vi "Acquire.vi"(5 "Cluster in":T1={"Queue Array"=[], "Queue Element"={"state"="", "data"=variant}, "System Event"=refnum, "System Event RefNum"=refnum, "Queue List"=[], "LPCA COM"="", "Rotating"=FALSE, "PrecorAI"="", "T_0 Index"=0, "Bar Graph X"=[], "Channels"=[], "Active Indicies"=[], "Active Channels"=[], "Sample Frequency"=0.0, "Ibrake Sweep"=[], "RPM Sweep"=[], "Load Sweep"=[], "Step Height Sweep"=[], "Range Sweep"=[], "A Counter"=0, "B Counter"=0, "C Counter"=0, "#A"=0, "#B"=0, "#C"=0, "Current RPM"=0.0, "Current Ibrake"=0, "Current Range"=0, "Current Step Height"=0, "Load Bank"=enum."OFF", "Cfg Cntrls"=[], "T_Monitor Indices"=[], "Thermal Limit"=0, "Thermal Resume"=0, "Timer Reset"=FALSE, "Stop Time"=0.0, "Autotest"=FALSE, "Pulsed RPM Capture"=FALSE, "Get Sample"=FALSE, "Last State"="", "Reset Timeout"=FALSE, "Ctrl Refs"={"Test Details"=refnum, "Save Config"=refnum, "Load Config"=refnum, "Path"=refnum, "Snapshot"=refnum, "SS#"=refnum, "Ibrake"=refnum, "RPM Target"=refnum, "Spin"=refnum, "Load Bank"=refnum, "Start Test"=refnum, "Pause Test"=refnum, "Load Sweep"=refnum, "RPM Sweep"=refnum, "Ibrake Sweep"=refnum, "Filters"=refnum, "Sample Frequency"=refnum, "Data Setup"=refnum, "Pause"=refnum, "Stop Time"=refnum, "S Period"=refnum, "Range"=refnum, "Step Height"=refnum, "Step Height Sweep"=refnum, "Range Sweep"=refnum, "Available Tests"=refnum, "RPM Graph"=refnum, "RPM Knob"=refnum, "FanMode"=refnum, "Fan Mode LED Array"=refnum, "Thermal Equilibrium"=refnum, "Data Display"=refnum, "LPCA Error"=refnum, "LPCA Ramp"=refnum, "LPCA Range"=refnum, "LPCA Resistance"=refnum, "Analyze Read"=refnum, "Console Select"=refnum, "Sub Panel"=refnum}, "Pulse Waveform"={"t0"=timestamp(0 s since 1904-01-01), "dt"=1.0, "Y"=[]}, "Snapshot"={"Test Details"="test", "Version"="test", "Date"=timestamp(3493915594.3018084 s since 1904-01-01), "Selected Test"="man", "Snapshot Number"=0, "Time"=timestamp(3493915602.7292905 s since 1904-01-01), "Ibrake Setpoint"="1", "RPM Setpoint"="20", "Range Setpoint"="", "Step Height Setpoint"="", "Load Bank Setpoint"="15", "Measurement Headers"="a,b,c,1,2,3", "Measurements"="1,2,3,4,5,6,7,8", "A"=0, "B"=0, "C"=0, "Raw Data"=[], "Available Tests"=enum."Manual", "Ibrake List"="", "RPM List"="", "Load Bank List"="", "Range List"="", "Step Height List"="", "FanMode Setpoint"=enum."Auto"}, "Sample Period"=0.0, "OverTemp"=FALSE, "Available Tests"=enum."Manual", "FanMode"=enum."Auto", "Fan Mode LED Array"=[FALSE, TRUE, FALSE], "Thermal\nEquilibrium "=FALSE, "Equilibrium Stop"=FALSE, "AvgDegChg"=[]} {"Snapshot"."Time" format="%<%H:%M:%S>T"; "Snapshot"."Date" format="%<%m/%d/%Y>T"}, 7 "Filters":T9(ring), 9 "Available Tests":T6, 10 "Active":bool, 11 "error in (no error)":errorcluster, 12 "Snapshot in":bool) -> (1 "output cluster":T1={"Queue Array"=[], "Queue Element"={"state"="", "data"=variant}, "System Event"=refnum, "System Event RefNum"=refnum, "Queue List"=[], "LPCA COM"="", "Rotating"=FALSE, "PrecorAI"="", "T_0 Index"=0, "Bar Graph X"=[], "Channels"=[], "Active Indicies"=[], "Active Channels"=[], "Sample Frequency"=0.0, "Ibrake Sweep"=[], "RPM Sweep"=[], "Load Sweep"=[], "Step Height Sweep"=[], "Range Sweep"=[], "A Counter"=0, "B Counter"=0, "C Counter"=0, "#A"=0, "#B"=0, "#C"=0, "Current RPM"=0.0, "Current Ibrake"=0, "Current Range"=0, "Current Step Height"=0, "Load Bank"=enum."OFF", "Cfg Cntrls"=[], "T_Monitor Indices"=[], "Thermal Limit"=0, "Thermal Resume"=0, "Timer Reset"=FALSE, "Stop Time"=0.0, "Autotest"=FALSE, "Pulsed RPM Capture"=FALSE, "Get Sample"=FALSE, "Last State"="", "Reset Timeout"=FALSE, "Ctrl Refs"={"Test Details"=refnum, "Save Config"=refnum, "Load Config"=refnum, "Path"=refnum, "Snapshot"=refnum, "SS#"=refnum, "Ibrake"=refnum, "RPM Target"=refnum, "Spin"=refnum, "Load Bank"=refnum, "Start Test"=refnum, "Pause Test"=refnum, "Load Sweep"=refnum, "RPM Sweep"=refnum, "Ibrake Sweep"=refnum, "Filters"=refnum, "Sample Frequency"=refnum, "Data Setup"=refnum, "Pause"=refnum, "Stop Time"=refnum, "S Period"=refnum, "Range"=refnum, "Step Height"=refnum, "Step Height Sweep"=refnum, "Range Sweep"=refnum, "Available Tests"=refnum, "RPM Graph"=refnum, "RPM Knob"=refnum, "FanMode"=refnum, "Fan Mode LED Array"=refnum, "Thermal Equilibrium"=refnum, "Data Display"=refnum, "LPCA Error"=refnum, "LPCA Ramp"=refnum, "LPCA Range"=refnum, "LPCA Resistance"=refnum, "Analyze Read"=refnum, "Console Select"=refnum, "Sub Panel"=refnum}, "Pulse Waveform"={"t0"=timestamp(0 s since 1904-01-01), "dt"=1.0, "Y"=[]}, "Snapshot"={"Test Details"="test", "Version"="test", "Date"=timestamp(3493915594.3018084 s since 1904-01-01), "Selected Test"="man", "Snapshot Number"=0, "Time"=timestamp(3493915602.7292905 s since 1904-01-01), "Ibrake Setpoint"="1", "RPM Setpoint"="20", "Range Setpoint"="", "Step Height Setpoint"="", "Load Bank Setpoint"="15", "Measurement Headers"="a,b,c,1,2,3", "Measurements"="1,2,3,4,5,6,7,8", "A"=0, "B"=0, "C"=0, "Raw Data"=[], "Available Tests"=enum."Manual", "Ibrake List"="", "RPM List"="", "Load Bank List"="", "Range List"="", "Step Height List"="", "FanMode Setpoint"=enum."Auto"}, "Sample Period"=0.0, "OverTemp"=FALSE, "Available Tests"=enum."Manual", "FanMode"=enum."Auto", "Fan Mode LED Array"=[FALSE, TRUE, FALSE], "Thermal\nEquilibrium "=FALSE, "Equilibrium Stop"=FALSE, "AvgDegChg"=[]} {"Snapshot"."Time" format="%<%H:%M:%S>T"; "Snapshot"."Date" format="%<%m/%d/%Y>T"}, 3 "Over Temp":bool, 4 "Heartbeat":bool caption="Time has Elapsed", 6 "Parsed Data":T8, 8 "Mean RPM":dbl format="%0.2f", 13 "RPM Wfm":cluster{"X":dbl, "Y":dbl}[](array[cluster]), 14 "Waveform 5 seconds":waveform(dbl)[](array[waveform]), 15 "error out":errorcluster)   [LabVIEW 2017]
uses:
  Controls/Available Tests.ctl
  Controls/Test TypeDef.ctl
  Code Library/Queue References Array.ctl
  Code Library/Queue Element.ctl
  Controls/Load Bank.ctl
  Console Sim/Controls/Console Select.ctl
  Controls/Snapshot Typedef.ctl
  Controls/FanMode.ctl
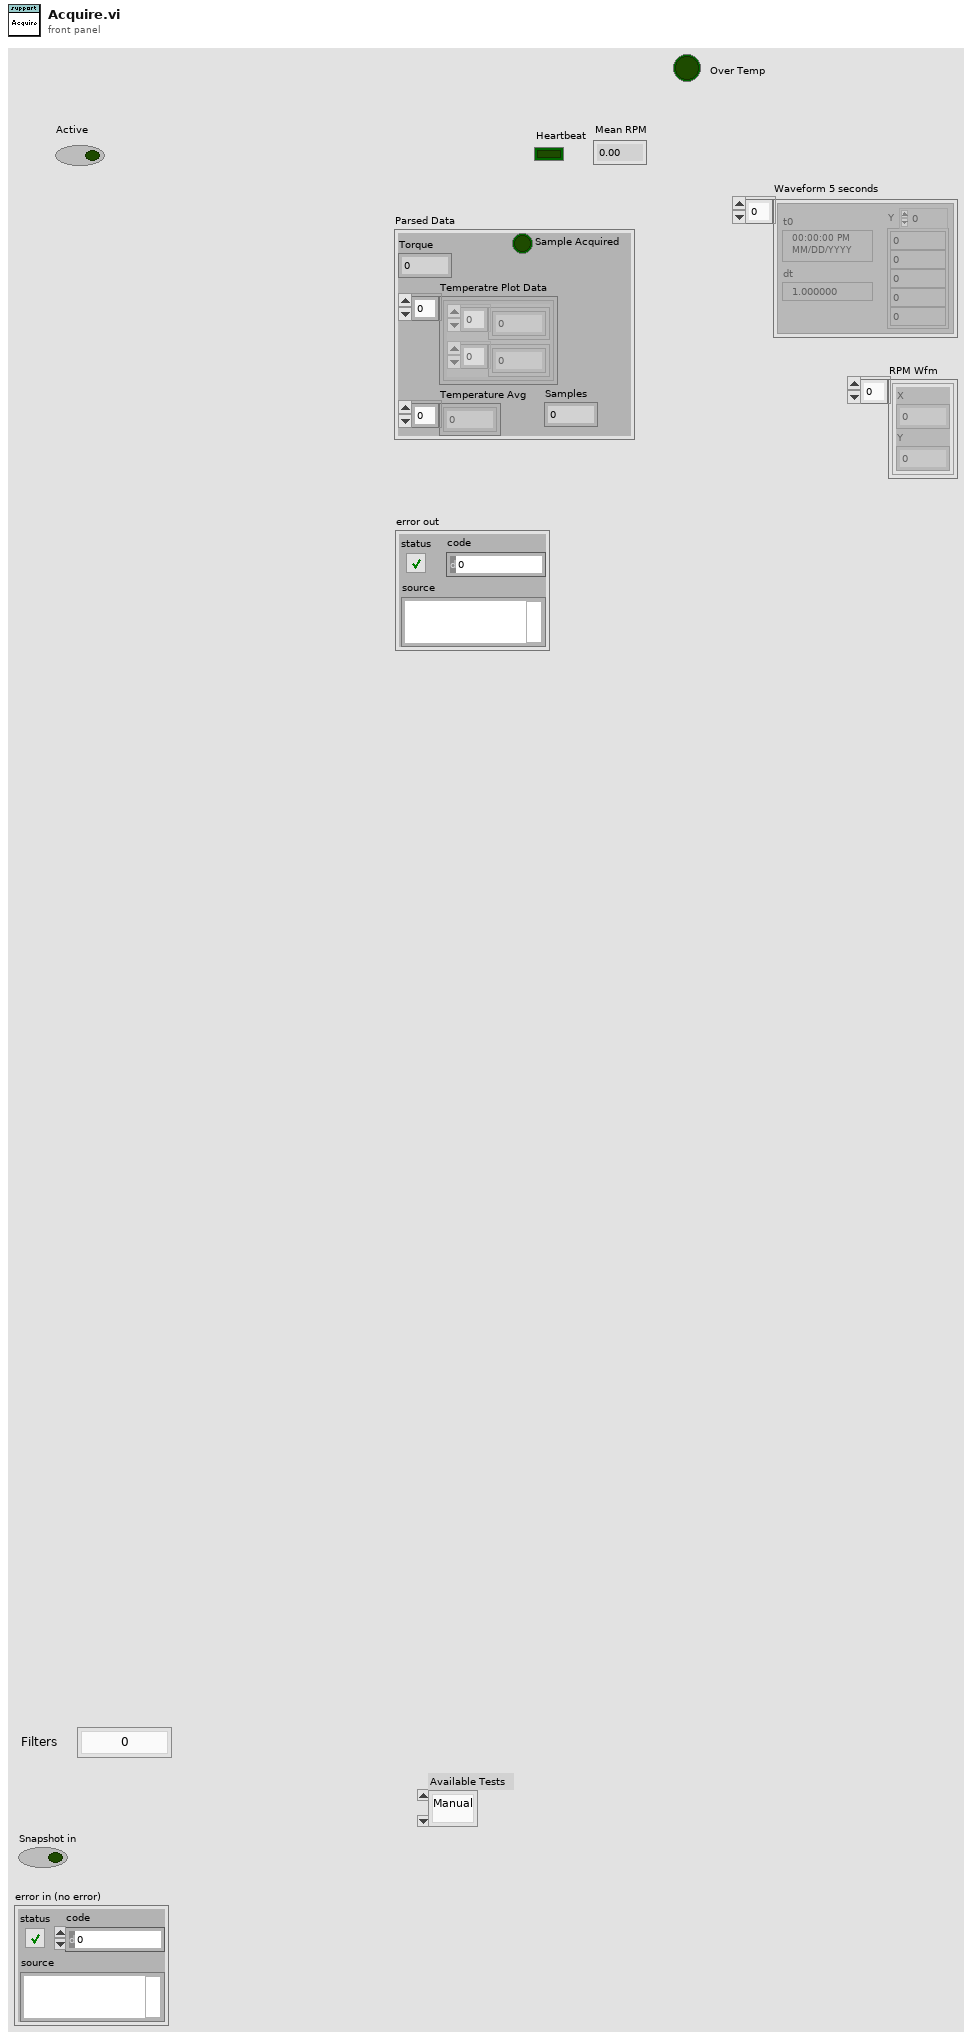
[diagram p1: front panel]
types:
  T1 = typedef "Test TypeDef.ctl" = cluster{"Queue Array":T2, "Queue Element":T3, "System Event":refnum<user-event>, "System Event RefNum":refnum<event-registration>, "Queue List":string[], "LPCA COM":refnum<visa-resource-name>, "Rotating":bool, "PrecorAI":refnum<k21>, "T_0 Index":i32, "Bar Graph X":i32[], "Channels":string[], "Active Indicies":i32[], "Active Channels":string[][], "Sample Frequency":dbl, "Ibrake Sweep":string[], "RPM Sweep":string[], "Load Sweep":string[], "Step Height Sweep":string[], "Range Sweep":string[], "A Counter":i32, "B Counter":i32, "C Counter":i32, "#A":i32, "#B":i32, "#C":i32, "Current RPM":dbl, "Current Ibrake":u32, "Current Range":u32, "Current Step Height":u32, "Load Bank":T4, "Cfg Cntrls":refnum<vi>[], "T_Monitor Indices":i32[], "Thermal Limit":i32, "Thermal Resume":i32, "Timer Reset":bool, "Stop Time":dbl, "Autotest":bool, "Pulsed RPM Capture":bool, "Get Sample":bool, "Last State":string, "Reset Timeout":bool, "Ctrl Refs":cluster{"Test Details":refnum<vi>, "Save Config":refnum<vi>, "Load Config":refnum<vi>, "Path":refnum<vi>, "Snapshot":refnum<vi>, "SS#":refnum<vi>, "Ibrake":refnum<vi>, "RPM Target":refnum<vi>, "Spin":refnum<vi>, "Load Bank":refnum<vi>, "Start Test":refnum<vi>, "Pause Test":refnum<vi>, "Load Sweep":refnum<vi>, "RPM Sweep":refnum<vi>, "Ibrake Sweep":refnum<vi>, "Filters":refnum<vi>, "Sample Frequency":refnum<vi>, "Data Setup":refnum<vi>, "Pause":refnum<vi>, "Stop Time":refnum<vi>, "S Period":refnum<vi>, "Range":refnum<vi>, "Step Height":refnum<vi>, "Step Height Sweep":refnum<vi>, "Range Sweep":refnum<vi>, "Available Tests":refnum<vi>, "RPM Graph":refnum<vi>, "RPM Knob":refnum<vi>, "FanMode":refnum<vi>, "Fan Mode LED Array":refnum<vi>, "Thermal Equilibrium":refnum<vi>, "Data Display":refnum<vi>, "LPCA Error":refnum<vi>, "LPCA Ramp":refnum<vi>, "LPCA Range":refnum<vi>, "LPCA Resistance":refnum<vi>, "Analyze Read":refnum<vi>, "Console Select":refnum<vi>, "Sub Panel":refnum<vi>}, "Pulse Waveform":waveform(dbl), "Snapshot":T5, "Sample Period":dbl, "OverTemp":bool, "Available Tests":T6, "FanMode":T7, "Fan Mode LED Array":bool[], "Thermal\nEquilibrium ":bool, "Equilibrium Stop":bool, "AvgDegChg":dbl[]}
  T2 = typedef "Queue References Array.ctl" = refnum<queue>[]
  T3 = typedef "Queue Element.ctl" = cluster{"state":string, "data":variant}
  T4 = typedef "Load Bank.ctl" = enum16{"OFF", "50", "25", "16.7", "12.5", "10.0", "8.3", "7.1", "6.3", "5.6", "5.0", "4.5", "4.2", "3.8", "3.6", "3.3", "3.1"}
  T5 = typedef "Snapshot Typedef.ctl" = cluster{"Test Details":string, "Version":string, "Date":timestamp, "Selected Test":string, "Snapshot Number":u16, "Time":timestamp, "Ibrake Setpoint":string, "RPM Setpoint":string, "Range Setpoint":string, "Step Height Setpoint":string, "Load Bank Setpoint":string, "Measurement Headers":string, "Measurements":string, "A":i32, "B":i32, "C":i32, "Raw Data":string[][], "Available Tests":T6, "Ibrake List":string, "RPM List":string, "Load Bank List":string, "Range List":string, "Step Height List":string, "FanMode Setpoint":T7}
  T6 = typedef "Available Tests.ctl" = enum16{"Manual", "EFX Brake Torque", "Generator Torque", "EFX Brake Thermal", "Generator Thermal", "Pulsed RPM", "AMT Brake Torque", "Bike Brake Torque", "AMT Brake Thermal", "Bike Brake Thermal"}
  T7 = typedef "FanMode.ctl" = enum16{"On", "Off", "Auto"}
  T8 = cluster{"Sample Acquired":bool, "Torque":dbl, "Temperatre Plot Data":cluster{dbl[], i32[]}[], "Temperature Avg":dbl[], "Samples":i32}
  T9 = enum16{"0", "0.1", "0.2", "0.5", "1", "2", "5", "10", "20", "50", "100", "200", "500", "1000", "2000", "5000", "10000"}
  T10 = cluster{bool, "Torque":dbl, "Temperatre Plot Data":cluster{dbl[], i32[]}[], "Temperature Avg":dbl[], "number of samples per channel":i32}
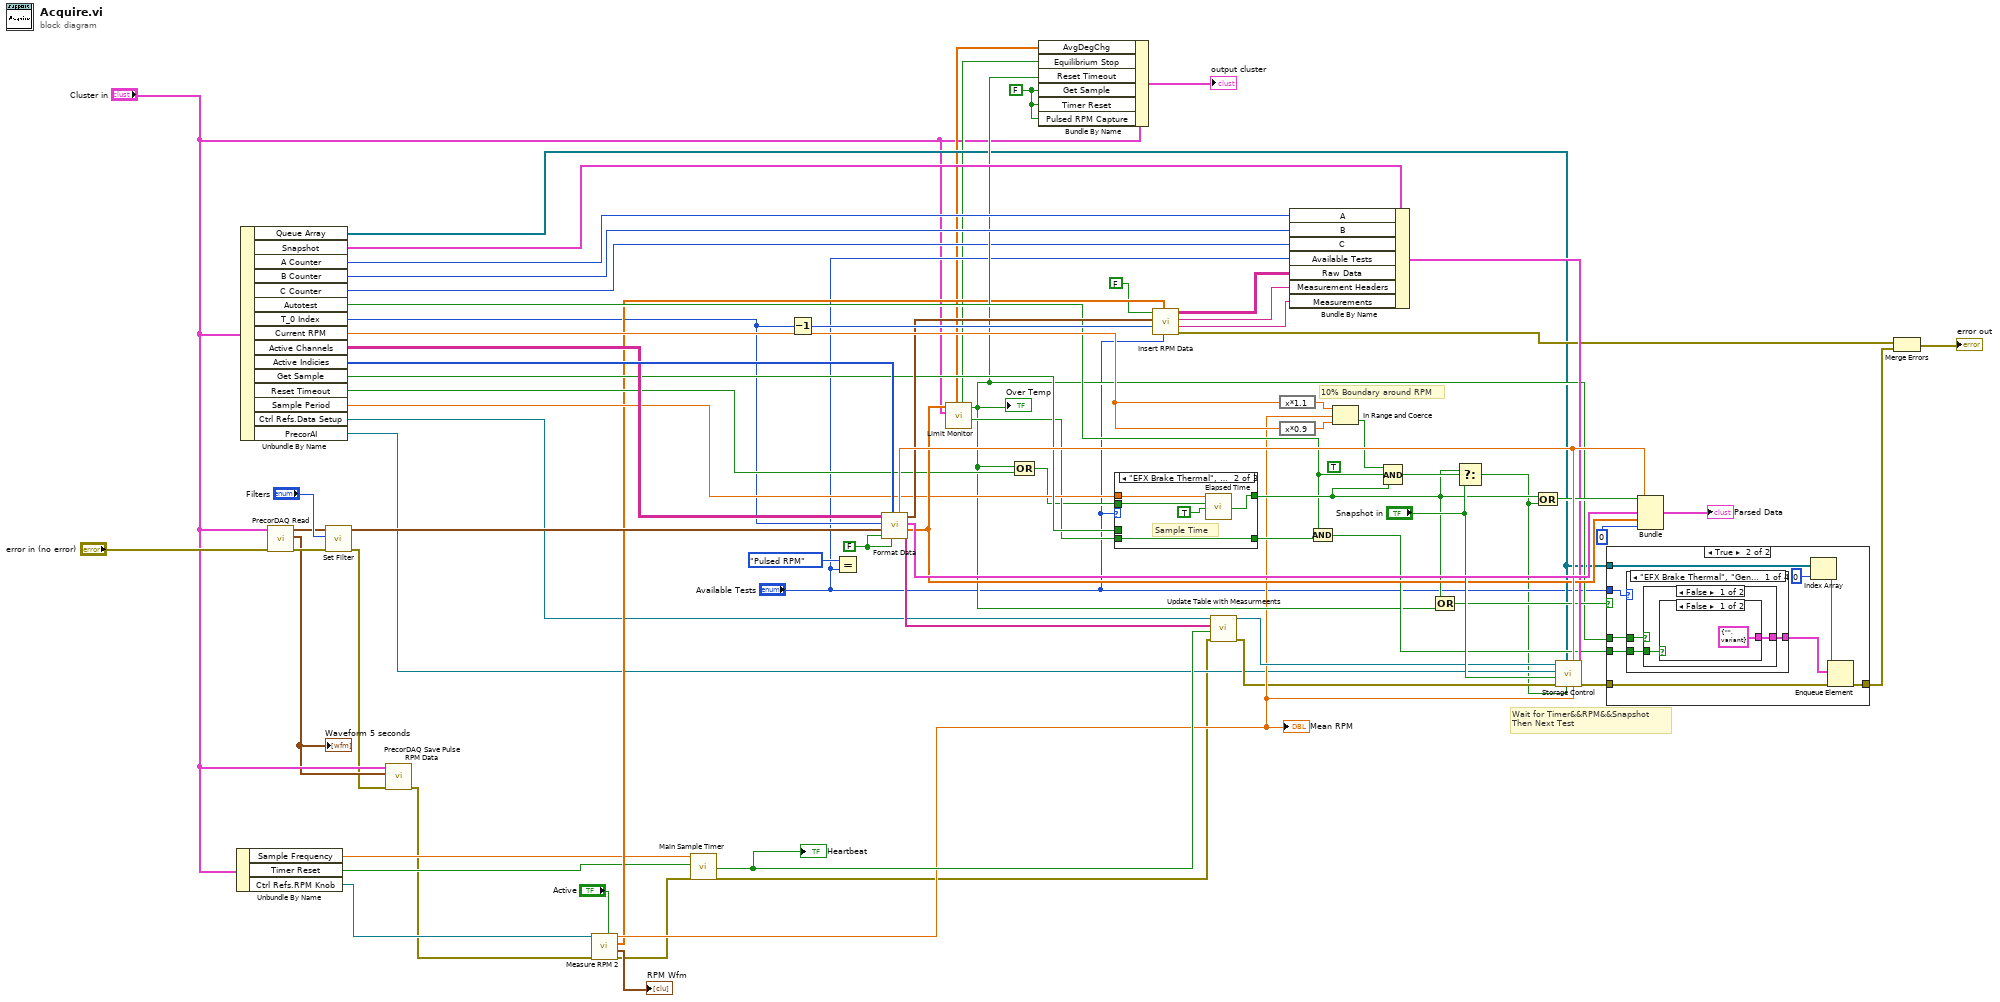
[diagram p0: block diagram]
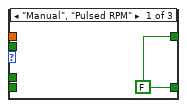
[diagram p2: hidden frame]
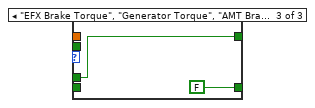
[diagram p3: hidden frame]
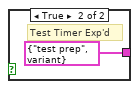
[diagram p5: hidden frame]
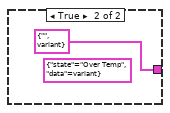
[diagram p6: hidden frame]
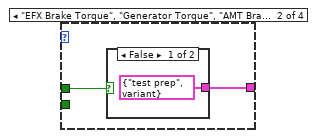
[diagram p7: hidden frame]
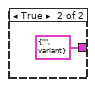
[diagram p8: hidden frame]
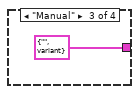
[diagram p9: hidden frame]
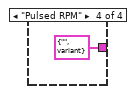
[diagram p10: hidden frame]
diagram:
  (unwired) TRUE ("value")
  w2 = FALSE ("Reset")
  w8 = FALSE
  # "10% Boundary around RPM"
  # "Wait for Timer&&RPM&&Snapshot\nThen Next Test"
  n1 = Unbundle By Name("Cluster in") -> ("Sample Frequency"=w11:dbl, "Timer Reset"=w12:bool, "Ctrl Refs.RPM Knob"=w16:refnum<vi>)
  n2 = Unbundle By Name("Cluster in") -> ("Queue Array"=w25:T2, "Snapshot"=w45:T5, "A Counter"=w56:i32, "B Counter"=w57:i32, "C Counter"=w33:i32, "Autotest"=w37:bool, "T_0 Index"=w22:i32, "Current RPM"=w65:dbl, "Active Channels"=w67:string[][], "Active Indicies"=w71:i32[], "Get Sample"=w50:bool, "Reset Timeout"=w36:bool, "Sample Period"=w43:dbl, "Ctrl Refs.Data Setup"=w28:refnum<vi>, "PrecorAI"=w13:refnum<k21>)
  n3 = call "PrecorDAQ Read.vi"("error in (no error)"="error in (no error)", "Cluster"="Cluster in") -> ("error out"=w15:errorcluster, "Data 5 seconds"=w6:waveform(dbl)[], "Data"=w14:waveform(dbl)[])  [unwired: 7 in]
  "Waveform 5 seconds" <- w6
  n4 = call "Set Filter.vi"("error in (no error)"=w15, "Filters"="Filters", "data"=w14) -> ("error out"=w5:errorcluster, "Array of Waveform"=w54:waveform(dbl)[])  [unwired: 7 in]
  n5 = call "PrecorDAQ Save Pulse RPM Data.vi"("error in (no error)"=w5, "Pulse RPM Data"=w6, "Cluster"="Cluster in") -> ("error out"=w4:errorcluster)  [unwired: 8 in]
  n6 = call "Measure RPM 2.vi"("Active"="Active", "error in"=w4, "Knob in"=w16) -> ("error out"=w10:errorcluster, "RPM Wfm"=→"RPM Wfm":cluster{"X":dbl, "Y":dbl}[], "Raw"=w30:dbl[], "Median RPM"=w31:dbl)  [unwired: 5 in]
  "Mean RPM" <- w31
  n7 = call "Main Sample Timer"("Time Target (s)"=w11, "Reset"=w12, "error in (no error)"=w10) -> ("Time has Elapsed"=w51:bool, "error out"=w9:errorcluster)  [unwired: 9 in, 6 out]
  "Heartbeat" <- w51
  n8 = Decrement(x=w22) -> (x-1=w55:i32)
  n9 = Equal?(x=Available_Tests."Pulsed RPM", y="Available Tests") -> ()  [unwired: 1 out]
  n10 = call "Format Data.vi"("Raw?"=w2, "Inidicies"=w71, "Reset"=w2, "data"=w54, "T_0 Index"=w22, "Active Channels"=w67) -> ("AI Chan Avg."=w68:string[], "Temperature Avg"=w61:dbl[], "Temperatre Plot Data"=w74:cluster{dbl[], i32[]}[], "Data Out"=w53:waveform(dbl)[], "Torque"=w62:dbl)  [unwired: 1 out]
  n11 = call "Limit Monitor.vi"("Cluster"="Cluster in", "Temperature Avg"=w61) -> ("Test Timer"=w41:bool, "Over Temp"=w34:bool, "Equilibrium Stop"=w20:bool, "AvgDegChg"=w19:dbl[])  [unwired: 6 in]
  "Over Temp" <- w34
  n12 = Compound Arithmetic op=OR(w34, w36) -> (w35:bool)
  n13 = Bundle By Name(cluster="Cluster in", "AvgDegChg"=w19, "Equilibrium Stop"=w20, "Reset Timeout"=w34, "Get Sample"=w8, "Timer Reset"=w8, "Pulsed RPM Capture"=w8) -> (→"output cluster":T1)
  n14 = case shown="\"EFX Brake Thermal\", \"Generator Thermal\", \"AMT Brake Thermal\", \"Bike Brake Thermal\"" "Available Tests" {
    tunnel: [w75 w79 w82] -> w42
    tunnel: w50 -> [_ _ w82]
    tunnel: w35 -> [_ w76 _]
    tunnel: w43 -> [_ w78 _]
    tunnel: w41 -> [_ w77 _]
    tunnel: [w75 w77 FALSE ("Test Timer")] -> w39
    frame "Manual", "Pulsed RPM" {
      w75 = FALSE ("Test Timer")
    }
    frame "EFX Brake Thermal", "Generator Thermal", "AMT Brake Thermal", "Bike Brake Thermal" {
      # "Sample Time"
      n15 = call "Elapsed Time"("Time Target (s)"=w78, "Reset"=w76, "Auto Reset"=TRUE) -> ("Time has Elapsed"=w79:bool)  [unwired: 9 in, 7 out]
    }
    frame "EFX Brake Torque", "Generator Torque", "AMT Brake Torque", "Bike Brake Torque" {
    }
  }
  n16 = call "Insert RPM Data.vi"("Available Tests"="Available Tests", "Raw"=w30, "Numeric"=w55, "Data Out in"=w53, "Pulsed RPM Capture"=FALSE) -> ("error out"=w52:errorcluster, "Measurements"=w23:string, "Header"=w26:string, "Data Out out"=w24:string[][])  [unwired: 2 in, 1 out]
  n17 = call "Update Table with Measurmeents.vi"("error in (no error)"=w9, "Sample"=w51, "AI Chan Avg."=w68, "MulticolumnListbox in"=w28) -> ("error out"=w27:errorcluster, "MulticolumnListbox out"=w69:refnum<vi>)  [unwired: 6 in]
  n18 = expression code="x*1.1"(w65) -> (w63:dbl)
  n19 = expression code="x*0.9"(w65) -> (w64:dbl)
  n20 = Bundle By Name(cluster=w45, "A"=w56, "B"=w57, "C"=w33, "Available Tests"="Available Tests", "Raw Data"=w24, "Measurement Headers"=w26, "Measurements"=w23) -> (w58:T5)
  n21 = Compound Arithmetic op=AND(w37, w39) -> (w38:bool)
  n22 = In Range and Coerce(upper limit=w63, x=w31, lower limit=w64) -> (In Range?=w18:bool)  [unwired: 1 out]
  n23 = Compound Arithmetic op=AND(w18, w37, w42) -> (w44:bool)
  n24 = Compound Arithmetic op=OR(w42, w34) -> (w40:bool)
  n25 = Select(t=w42, s=w44, f="Snapshot in") -> (s? t:f=w1:bool)
  n26 = Compound Arithmetic op=OR(w42, w1) -> (w60:bool)
  n27 = call "Storage Control.vi"(3:"Snapshot"=w58, "RPM"=w31, "Torque"=w62, 6:"Snapshot"=w1, "Queue Array"=w25, "error in (no error)"=w27, "Manual Snapshot"="Snapshot in", "task in"=w13, "MulticolumnListbox in"=w69) -> ("error out"=w66:errorcluster)  [unwired: 2 in]
  n28 = case shown="True" w40 {
    tunnel: w66 -> [w83 w92]
    tunnel: [w83 w91] -> w47
    tunnel: w25 -> [_ w90]
    tunnel: w34 -> [_ w87]
    tunnel: w38 -> [_ w84]
    tunnel: "Available Tests" -> [_ w85]
    frame False {
    }
    frame True {
      n29 = case shown="\"EFX Brake Thermal\", \"Generator Thermal\", \"AMT Brake Thermal\", \"Bike Brake Thermal\"" w85 {
        tunnel: w87 -> [w95 w101 _ _]
        tunnel: [w94 w102 T3 {"state"="", "data"=variant} ("element") T3 {"state"="", "data"=variant} ("element")] -> w86
        tunnel: w84 -> [w93 _ _ _]
        frame "EFX Brake Thermal", "Generator Thermal", "AMT Brake Thermal", "Bike Brake Thermal" {
          n30 = case shown="False" w95 {
            tunnel: [w96 T3 {"state"="", "data"=variant} ("element")] -> w94
            tunnel: w93 -> [w97 _]
            frame False {
              n31 = case shown="False" w97 {
                tunnel: [T3 {"state"="", "data"=variant} ("element") T3 {"state"="test prep", "data"=variant} ("element")] -> w96
                frame False {
                }
                frame True {
                  # "Test Timer Exp'd"
                }
              }
            }
            frame True {
              (unwired) T3 {"state"="Over Temp", "data"=variant} ("element")
            }
          }
        }
        frame "EFX Brake Torque", "Generator Torque", "AMT Brake Torque", "Bike Brake Torque" {
          n32 = case shown="False" w101 {
            tunnel: [T3 {"state"="test prep", "data"=variant} ("element") T3 {"state"="", "data"=variant} ("element")] -> w102
            frame False {
            }
            frame True {
            }
          }
        }
        frame "Manual" {
        }
        frame "Pulsed RPM" {
        }
      }
      n33 = Index Array(array=w90, index=0) -> (element=w88:refnum<queue>)
      n34 = Enqueue Element(queue=w88, element=w86, error in (no error)=w92) -> (error out=w91:errorcluster)  [unwired: 1 in, 2 out]
    }
  }
  n35 = Bundle(w60, "Torque"=w62, "Temperatre Plot Data"=w74, "Temperature Avg"=w61, "number of samples per channel"=0) -> (→"Parsed Data":T10)  [unwired: 1 in]
  n36 = Merge Errors(w52, w47) -> (→"error out":errorcluster)
